vi "前面板控件引用剔除.vi"(10 "数组":string[](array[string]), 11 "VI输入":refnum<vi>) -> (2 "已删除控件":refnum<vi>[](array[refnum]), 3 "删除后控件":refnum<vi>[](array[refnum]))   [LabVIEW 2017]
panel:
  out "数组 5":i32[](array[numeric])
  out "数组 4":string[](array[string])
  out "数组 3":string[](array[string])
  out "数组 2":string[](array[string])
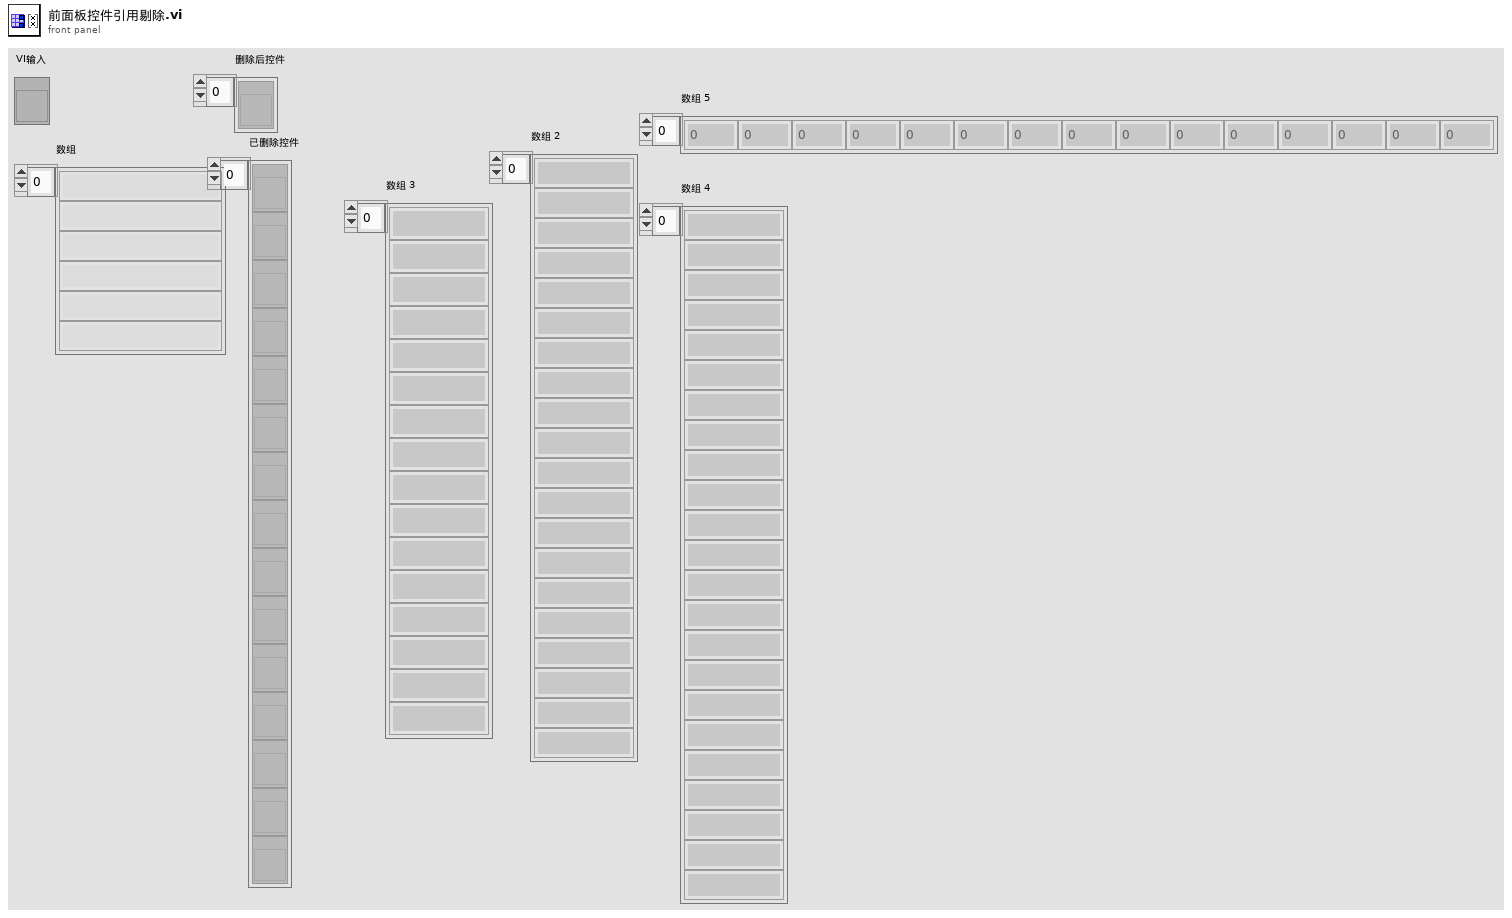
[diagram p1: front panel]
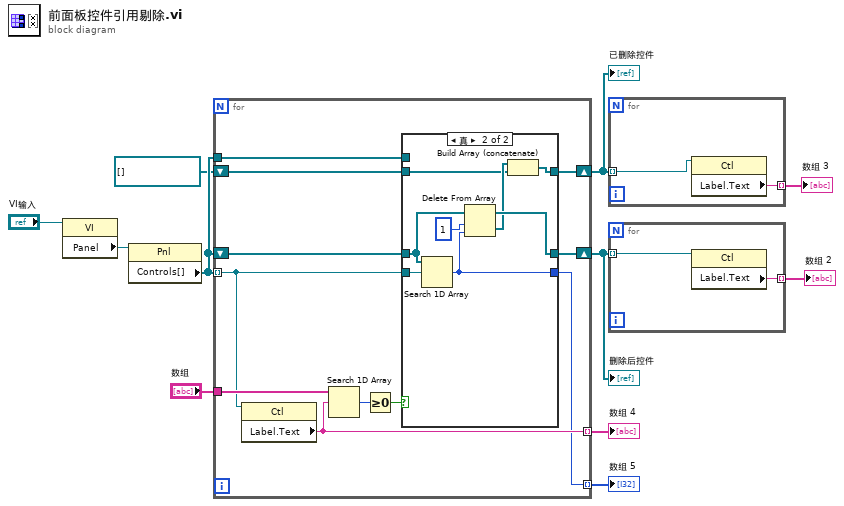
[diagram p0: block diagram]
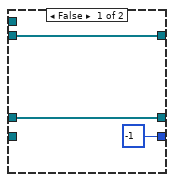
[diagram p2: hidden frame]
diagram:
  n1 = property on="属性节点" class="VI"(reference="VI输入") -> ("Panel"=w10:refnum<vi>)  [unwired: 1 in, 2 out]
  n2 = property on="属性节点" class="Pnl"(reference=w10) -> ("Controls[]"=w4:refnum<vi>[])  [unwired: 1 in, 2 out]
  n3 = for {
    tunnel: w4 -> [w12] mode=indexing
    tunnel: "数组" -> [w22]
    shift-right: [w18] -> w8
    shift-left: w4 -> [w20]
    shift-right: [w16] -> w6
    shift-left: refnum<vi>[] [] -> [w17]
    tunnel: w4 -> [w15]
    tunnel: [w14] -> w3 mode=indexing
    tunnel: [w13] -> w2 mode=indexing
    n4 = property class="Ctl"(reference=w12) -> ("Label.Text"=w14:string)  [unwired: 1 in, 2 out]
    n5 = Search 1D Array(1D array=w22, element=w14) -> (index of element=w21:i32)  [unwired: 1 in]
    n6 = Greater Or Equal To 0?(x=w21) -> (x >= 0?=w19:bool)
    n7 = case shown="真" w19 {
      tunnel: w20 -> [w25 w28]
      tunnel: [w25 w32] -> w18
      tunnel: w17 -> [w24 w30]
      tunnel: [w24 w29] -> w16
      tunnel: w15 -> [_ _]
      tunnel: [-1 w26] -> w13
      tunnel: w12 -> [_ w27]
      frame False {
      }
      frame True {
        n8 = Search 1D Array(1D array=w28, element=w27) -> (index of element=w26:i32)  [unwired: 1 in]
        n9 = Delete From Array(array=w28, length=1 ("长度"), index=w26) -> (deleted portion=w31:refnum<vi>[], array with subset deleted=w32:refnum<vi>[])
        n10 = Build Array (concatenate)(w31, w30) -> (w29:refnum<vi>[])
      }
    }
  }
  "删除后控件" <- w8
  "已删除控件" <- w6
  "数组 4" <- w3
  "数组 5" <- w2
  n11 = for {
    tunnel: w6 -> [w35] mode=indexing
    tunnel: [w34] -> w5 mode=indexing
    n12 = property class="Ctl"(reference=w35) -> ("Label.Text"=w34:string)  [unwired: 1 in, 2 out]
  }
  "数组 3" <- w5
  n13 = for {
    tunnel: w8 -> [w37] mode=indexing
    tunnel: [w36] -> w7 mode=indexing
    n14 = property class="Ctl"(reference=w37) -> ("Label.Text"=w36:string)  [unwired: 1 in, 2 out]
  }
  "数组 2" <- w7
